vi "PERTRAS Initialisierung.vi"() -> ()   [LabVIEW 2010]
uses:
  <vilib>/Utility/error.llb/DialogType.ctl
  <vilib>/Instr/_visa.llb/VISA Configure Serial Port (Instr).vi
panel:
  in  "Messwerte speichern":path
  in  "Pfad ändern?":bool
  in  "anderen Speicherpfad wählen?":path
  out "Fluss-/Druckregler Block1":bool
  out "Multipositionsventil":bool
  in  "andere Konfigurationsdatei wählen?":path
  in  "andere Konfig.-Datei wählen?":bool
  in  "Konfigurationsdatei":path
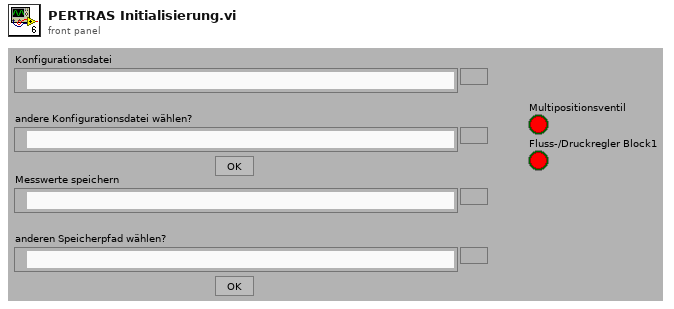
[diagram p1: front panel]
types:
  T1 = enum16{"open", "replace", "create", "open or create", "replace or create", "replace or create with confirmation"}
  T2 = typedef "DialogType.ctl" = u16
  T3 = cluster{"Mode":enum16{"RTU", "ASCII"}, "Slave Address":u8}
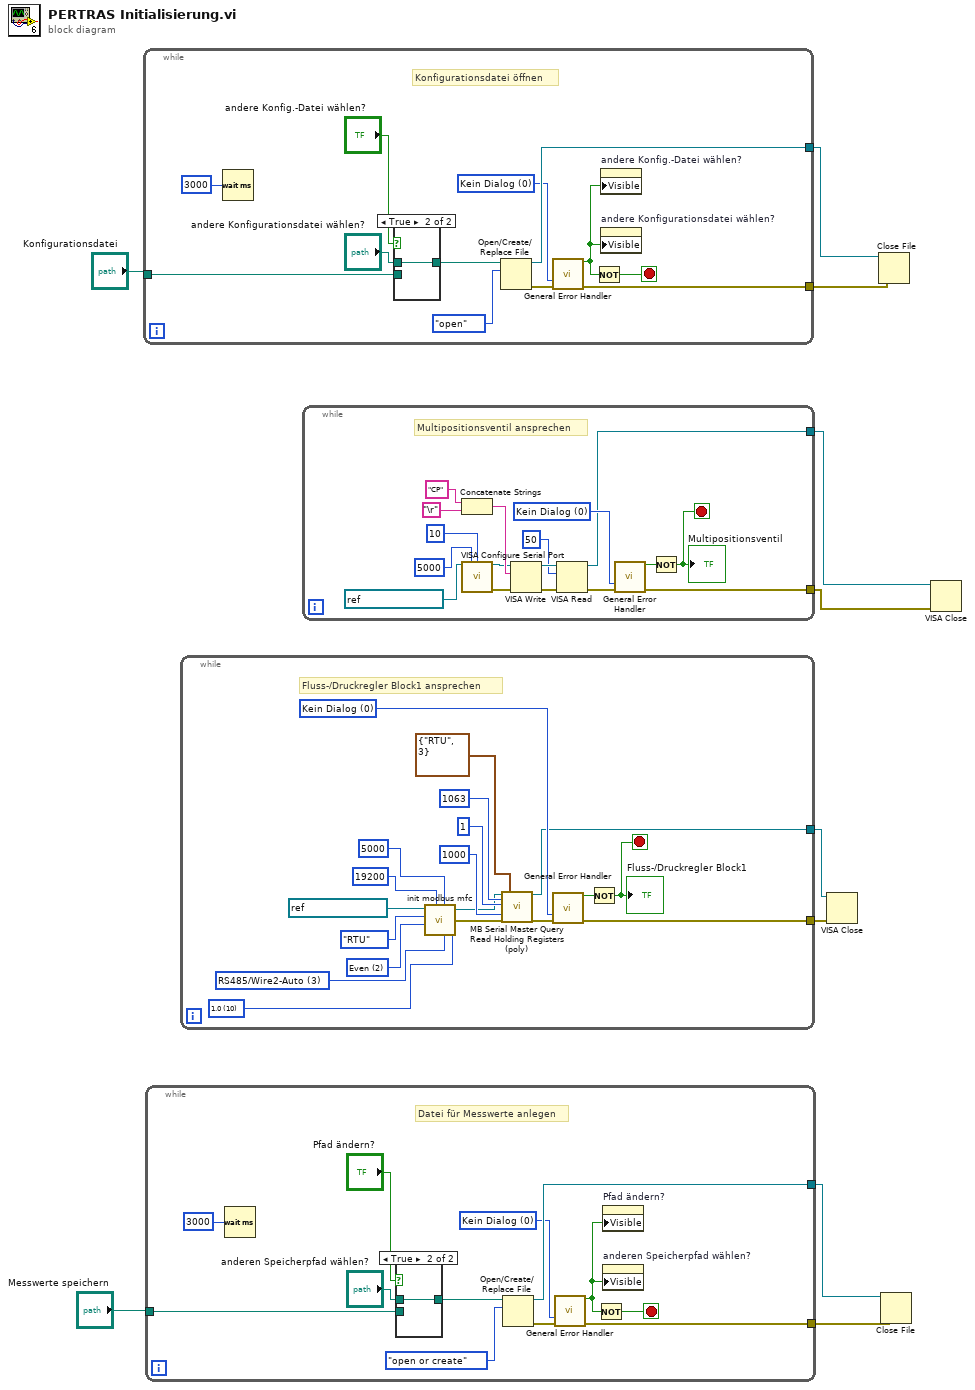
[diagram p0: block diagram]
diagram:
  n1 = while {
    tunnel: [w21] -> w9
    tunnel: [w17] -> w8
    tunnel: "Konfigurationsdatei" -> [w14]
    stop <- w19 stop-if-true
    w18 = T2 0 items=["Kein Dialog", "OK-Meldung", "Dialog zum Fortsetzen oder Anhalten", "OK-Meldung + Warnungen", "Weiter/Stopp + Warnung"] ("type of dialog (OK msg:1)")
    # "Konfigurationsdatei öffnen"
    n2 = Wait (ms)(milliseconds to wait=u32 3000 ("Zu wartende ms")) -> ()  [unwired: 1 out]
    n3 = case shown="True" "andere Konfig.-Datei wählen?" {
      tunnel: w14 -> [w23 _]
      tunnel: [w23 w24] -> w13
      tunnel: "andere Konfigurationsdatei wählen?" -> [_ w24]
      frame False {
      }
      frame True {
      }
    }
    n4 = Open/Create/Replace File(file path (use dialog)=w13, operation (0:open)=T1."open" ("Operation (0:Öffnen)")) -> (refnum out=w21:refnum<file>, error out=w20:errorcluster)  [unwired: 4 in, 1 out]
    n5 = call <vilib>:"General Error Handler.vi"("type of dialog (OK msg:1)"=w18, "error in (no error)"=w20) -> ("error?"=w11:bool, "error out"=w17:errorcluster)  [unwired: 9 in, 3 out]
    n6 = Not(x=w11) -> (.not. x?=w19:bool)
    n7 = property on="andere Konfig.-Datei wählen?" class="Bool"("Visible"=w11) -> ()  [unwired: 2 in, 2 out]
    n8 = property on="andere Konfigurationsdatei wählen?" class="Path"("Visible"=w11) -> ()  [unwired: 2 in, 2 out]
  }
  n9 = while {
    tunnel: [w35] -> w2
    tunnel: [w31] -> w1
    tunnel: "Messwerte speichern" -> [w28]
    stop <- w33 stop-if-true
    w32 = T2 0 items=["Kein Dialog", "OK-Meldung", "Dialog zum Fortsetzen oder Anhalten", "OK-Meldung + Warnungen", "Weiter/Stopp + Warnung"] ("type of dialog (OK msg:1)")
    # "Datei für Messwerte anlegen"
    n10 = Wait (ms)(milliseconds to wait=u32 3000 ("Zu wartende ms")) -> ()  [unwired: 1 out]
    n11 = case shown="True" "Pfad ändern?" {
      tunnel: w28 -> [w37 _]
      tunnel: [w37 w38] -> w27
      tunnel: "anderen Speicherpfad wählen?" -> [_ w38]
      frame False {
      }
      frame True {
      }
    }
    n12 = Open/Create/Replace File(file path (use dialog)=w27, operation (0:open)=T1."open or create" ("Operation (0:Öffnen)")) -> (refnum out=w35:refnum<file>, error out=w34:errorcluster)  [unwired: 4 in, 1 out]
    n13 = call <vilib>:"General Error Handler.vi"("type of dialog (OK msg:1)"=w32, "error in (no error)"=w34) -> ("error?"=w25:bool, "error out"=w31:errorcluster)  [unwired: 9 in, 3 out]
    n14 = Not(x=w25) -> (.not. x?=w33:bool)
    n15 = property on="Pfad ändern?" class="Bool"("Visible"=w25) -> ()  [unwired: 2 in, 2 out]
    n16 = property on="anderen Speicherpfad wählen?" class="Path"("Visible"=w25) -> ()  [unwired: 2 in, 2 out]
  }
  n17 = while {
    tunnel: [w40] -> w5
    tunnel: [w47] -> w4
    stop <- w48 stop-if-true
    w50 = T2 0 items=["Kein Dialog", "OK-Meldung", "Dialog zum Fortsetzen oder Anhalten", "OK-Meldung + Warnungen", "Weiter/Stopp + Warnung"] ("type of dialog (OK msg:1)")
    w57 = u16 10 items=["1.0"=10, "1.5"=15, "2.0"=20] ("Serial Settings:Stop Bits")
    w55 = u16 2 items=["None", "Odd", "Even", "Mark", "Space"] ("Parity")
    w56 = i16 3 items=["Unknown"=-1, "RS485/Wire4"=0, "RS485/Wire2-EchoDTR"=1, "RS485/Wire2-CtrlDTR"=2, "RS485/Wire2-Auto"=3, "RS232/DTE"=128, "RS232/DCE"=129, "RS232/AUTO"=130] ("Serial Settings:Wire Mode")
    # "Fluss-/Druckregler Block1 ansprechen"
    n18 = call "init modbus mfc.vi"("Timeout"=u32 5000, "Serial Settings:Stop Bits"=w57, "Serial Settings:Wire Mode"=w56, "Baud Rate"=u32 19200, "VISA resource name"=refnum<visa-resource-name> "ASRL2::INSTR", "Mode"=enum16{"RTU", "ASCII"}."RTU", "Parity"=w55) -> ("VISA resource name out"=w43:refnum<visa-resource-name>, "error out"=w42:errorcluster)  [unwired: 2 in]
    n19 = call "MB Serial Master Query Read Holding Registers (poly).vi"("VISA resource name"=w43, "Starting Address"=u16 1063, "Quantity"=u16 1, "Timeout"=u32 1000, "error in"=w42, "Serial Parameters"=T3 {"Mode"=enum."RTU", "Slave Address"=3}) -> ("VISA resource name out"=w40:refnum<visa-resource-name>, "error out"=w41:errorcluster)  [unwired: 10 in, 2 out]
    n20 = call <vilib>:"General Error Handler.vi"("type of dialog (OK msg:1)"=w50, "error in (no error)"=w41) -> ("error?"=w49:bool, "error out"=w47:errorcluster)  [unwired: 9 in, 3 out]
    n21 = Not(x=w49) -> (.not. x?=w48:bool)
    "Fluss-/Druckregler Block1" <- w48
  }
  n22 = while {
    tunnel: [w71] -> w6
    tunnel: [w59] -> w7
    stop <- w73 stop-if-true
    w72 = T2 0 items=["Kein Dialog", "OK-Meldung", "Dialog zum Fortsetzen oder Anhalten", "OK-Meldung + Warnungen", "Weiter/Stopp + Warnung"] ("type of dialog (OK msg:1)")
    # "Multipositionsventil ansprechen"
    n23 = Concatenate Strings("CP" ("String"), "\r") -> (w65:string)
    n24 = call-poly "VISA Configure Serial Port"("VISA resource name"=refnum<visa-resource-name> "ASRL1::INSTR", "timeout (10sec)"=u32 5000, "termination char\n(0xA = '\\n' = LF)"=u8 10 ("termination char\n(0xA = '\\n' = LF)")) -> ("VISA resource name out"=w61:refnum<visa-resource-name>, "error out"=w60:errorcluster)  [unwired: 11 in]
    n25 = VISA Write(VISA resource name=w61, write buffer=w65, error in (no error)=w60) -> (VISA resource name out=w67:refnum<visa-resource-name>, error out=w66:errorcluster)  [unwired: 1 out]
    n26 = VISA Read(VISA resource name=w67, byte count=u32 50 ("Byte-Anzahl"), error in (no error)=w66) -> (VISA resource name out=w59:refnum<visa-resource-name>, error out=w58:errorcluster)  [unwired: 2 out]
    n27 = call <vilib>:"General Error Handler.vi"("type of dialog (OK msg:1)"=w72, "error in (no error)"=w58) -> ("error?"=w74:bool, "error out"=w71:errorcluster)  [unwired: 9 in, 3 out]
    n28 = Not(x=w74) -> (.not. x?=w73:bool)
    "Multipositionsventil" <- w73
  }
  n29 = VISA Close(VISA resource name=w5, error in (no error)=w4) -> ()  [unwired: 1 out]
  n30 = Close File(refnum=w9, error in=w8) -> ()  [unwired: 2 out]
  n31 = Close File(refnum=w2, error in=w1) -> ()  [unwired: 2 out]
  n32 = VISA Close(VISA resource name=w7, error in (no error)=w6) -> ()  [unwired: 1 out]
